vi "Stream Control (Inline).vi"(7 "future trigger":bool, 9 "input valid":bool, 11 "stream control":refnum<class "niUSRP Stream Control (DMA) v1 FPGA.lvclass">, 12 "ready for output":bool, 13 "trigger":bool) -> (4 "SPC - debug":u8, 10 "stream":bool, 14 "ready for input":bool, 15 "stream control":refnum<class "niUSRP Stream Control (DMA) v1 FPGA.lvclass">)   [LabVIEW 2025, in "niUSRP Stream Control (DMA) v1 FPGA.lvclass"]
uses:
  niUSRP Stream Control (DMA) v1 FPGA.lvclass
  niUSRP Stream Control (DMA) v1 FPGA.lvclass/niUSRP Stream Control (DMA) v1 FPGA.ctl
  <vilib>/rvi/eio/common/nirviEmuTemplateMethod_errors.vi
  <vilib>/rvi/DataTransferAndStorage/Container/Common/niFpgaContainerExecOnDevCompGetState.vi
  <vilib>/rvi/Emulation/niFpgaEmulationIsFPGAContextNoSignature.vi
  <vilib>/rvi/DataTransferAndStorage/Container/Common/niFpgaContainerGetUniqueNameForEmu.vi
  <vilib>/rvi/Memory/Memory_Emulation/niFpgaMemoryEmulationCacheClearOnFirstRun.vi
  <vilib>/rvi/Memory/Memory_Emulation/nirvimemoryEmulationManagerCache_MakeExclusive.vi
  <vilib>/rvi/Memory/Memory_Emulation/niFpgaMemoryEmulationValidateCache.vi
  <vilib>/rvi/Memory/Memory_Emulation/nirvimemoryEmulationManagerCache_InsertValue.vi
  <vilib>/Utility/error.llb/Clear Errors.vi
  <vilib>/rvi/Memory/Memory_Emulation/nirvimemoryEmulationManagerCache_ReleaseExclusive.vi
  <vilib>/rvi/Memory/Memory_Emulation/nirvimemoryEmulationManagerCache_GetValue.vi
  <vilib>/rvi/Memory/Memory_Emulation/nirvimemoryEmulationManagerCache_SetValue.vi
  <vilib>/rvi/Emulation/niFpgaProcessEmulError.vi
  <vilib>/rvi/Emulation/niFpgaSctlEmulationGetInTimedLoop.vi
  <vilib>/eio/EIONode/EIONode.xnode
  <vilib>/rvi/DataTransferAndStorage/Container/XNode/niFpgaContainer.xnode
  <vilib>/rvi/DataTransferAndStorage/Register/Emulation/niFpgaRegisterEmulationRefIn.vi
  <instrlib>/_niInstr/Basic Elements/v1/FPGA/niInstr Basic Elements v1 FPGA.lvlib
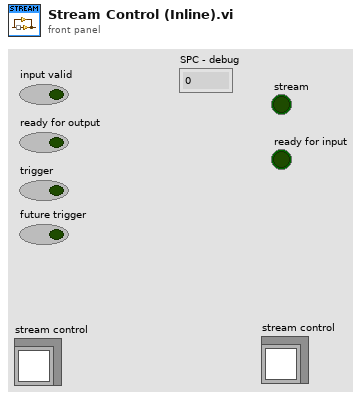
[diagram p1: front panel]
types:
  T1 = typedef "Stream Control State.ctl" = enum16{"Idle", "Active", "WaitForTrigger"}
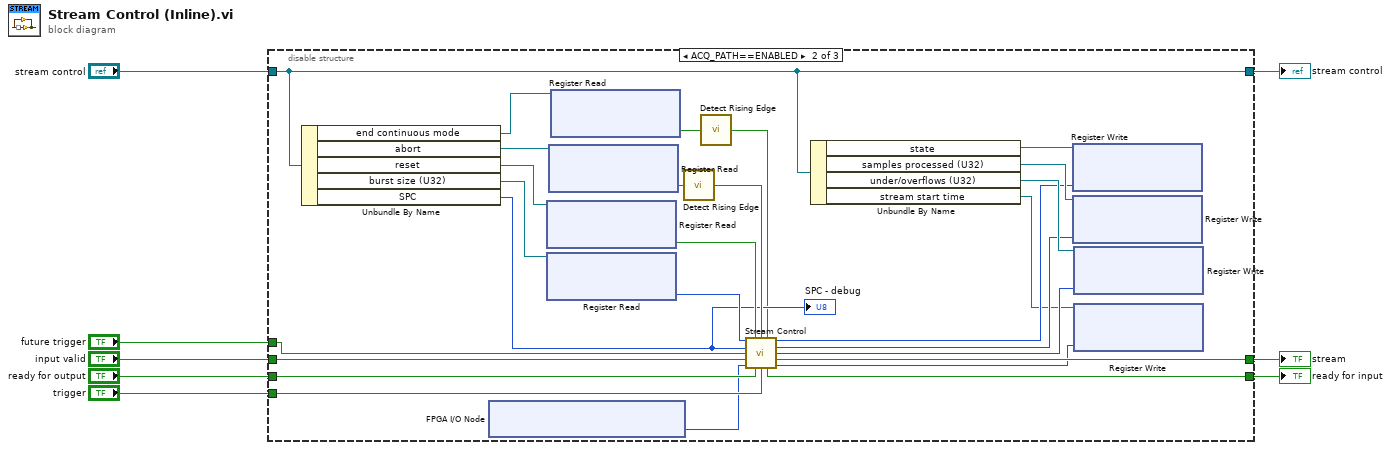
[diagram p0: block diagram]
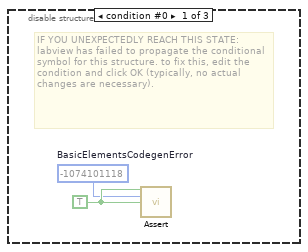
[diagram p2: hidden frame]
diagram:
  n1 = disable-structure shown="ACQ_PATH==ENABLED" {
    disable-tunnel: "input valid" -> [_ w27 _]
    disable-tunnel: "stream control" -> [_ w31 _]
    disable-tunnel: "ready for output" -> [_ w21 _]
    disable-tunnel: [_ w31 _] -> w5
    disable-tunnel: [_ w26 _] -> w4
    disable-tunnel: [_ w22 _] -> w3
    disable-tunnel: "trigger" -> [_ w29 _]
    disable-tunnel: "future trigger" -> [_ w11 _]
    frame condition #0 {
      w10 = TRUE ("assert")
      w9 = -1074101118  # BasicElementsCodegenError
      # "IF YOU UNEXPECTEDLY REACH THIS STATE:\nlabview has failed to propagate the conditional symbol for this structure. to fix this, edit the condition and click OK (typically, no actual changes are necessary)."
      n2 = call <instrlib>:"Assert.vi"("assert"=w10, "error code"=w9, "enable show error"=w10) -> ()  [unwired: 13 in]
    }
    frame condition #1 (active) {
      n3 = Unbundle By Name(w31) -> ("end continuous mode"=w17:refnum<k21>, "abort"=w19:refnum<k21>, "reset"=w36:refnum<k21>, "burst size (U32)"=w37:refnum<k21>, "SPC"=w18:u8)
      "SPC - debug" <- w18
      n4 = xnode "FPGA I/O Node"() -> ("Daughterboard 0\\Radio Time"=w12:u64)  [unwired: 1 in, 1 out]
      n5 = xnode ("Register Read")("Register In"=w36) -> ("Data"=w35:bool)  [unwired: 1 out]
      n6 = xnode ("Register Read")("Register In"=w37) -> ("Data"=w20:u32)  [unwired: 1 out]
      n7 = xnode ("Register Read")("Register In"=w19) -> ("Data"=w30:bool)  [unwired: 1 out]
      n8 = xnode ("Register Read")("Register In"=w17) -> ("Data"=w16:bool)  [unwired: 1 out]
      n9 = call <instrlib>:"Detect Rising Edge.vi"("signal"=w30) -> ("edge detected"=w28:bool)  [unwired: 14 in]
      n10 = call <instrlib>:"Detect Rising Edge.vi"("signal"=w16) -> ("edge detected"=w15:bool)  [unwired: 14 in]
      n11 = call "Stream Control.vi"("burst size"=w20, "reset"=w35, "abort"=w28, "end continuous mode"=w15, "samples per cycle (1)"=w18, "future trigger"=w11, "input valid"=w27, "current time"=w12, "fifo status"=w21, "start trigger"=w29) -> ("state"=w25:T1, "samples processed"=w24:u32, "number of malflows"=w23:u32, "stream"=w26:bool, "fifo ready"=w22:bool, "stream start time"=w13:u64)
      n12 = Unbundle By Name(w31) -> ("state"=w34:refnum<k21>, "samples processed (U32)"=w33:refnum<k21>, "under/overflows (U32)"=w32:refnum<k21>, "stream start time"=w14:refnum<k21>)
      n13 = xnode ("Register Write")("Data"=w25, "Register In"=w34) -> ()  [unwired: 1 out]
      n14 = xnode ("Register Write")("Data"=w24, "Register In"=w33) -> ()  [unwired: 1 out]
      n15 = xnode ("Register Write")("Data"=w23, "Register In"=w32) -> ()  [unwired: 1 out]
      n16 = xnode ("Register Write")("Data"=w13, "Register In"=w14) -> ()  [unwired: 1 out]
    }
    frame condition #2 {
    }
  }
  "stream control" <- w5
  "stream" <- w4
  "ready for input" <- w3
